vi "Agilent U2722 - Configure Chassis.vi"() -> ()   [LabVIEW 2018]
doc: "This VI shows how to configure chassis"
uses:
  <instrlib>/Agilent U2722/Agilent U2722.lvlib
panel:
  in  "Reference Clock Source (1: Auto)":i32(ring)=1 items=["Internal", "Auto"]
  in  "Trigger Out Bit (0)":i32
  in  "Chassis Identity (0)":i32
  in  "Chassis VISA resource name":refnum<visa-resource-name>
  # "(c) 2009-2015 National Instruments.  ALL RIGHTS RESERVED."
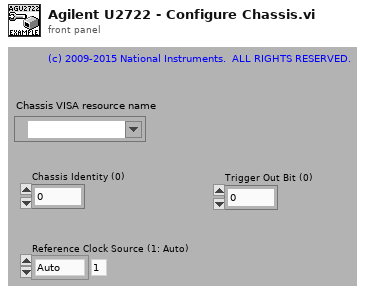
[diagram p1: front panel]
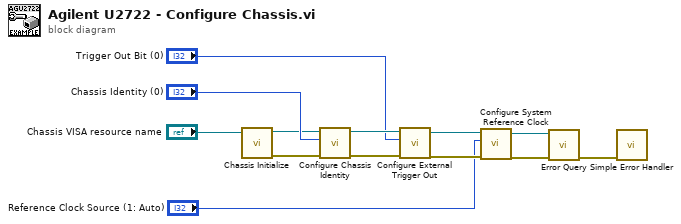
[diagram p0: block diagram]
diagram:
  n1 = call <instrlib>:"Chassis Initialize.vi"("Chassis VISA resource name"="Chassis VISA resource name") -> ("error out"=w2:errorcluster, "Chassis VISA resource name out"=w3:refnum<visa-resource-name>)  [unwired: 9 in]
  n2 = call <instrlib>:"Configure Chassis Identity.vi"("error in (no error)"=w2, "Chassis Identity (0)"="Chassis Identity (0)", "Chassis VISA resource name"=w3) -> ("error out"=w11:errorcluster, "Chassis VISA resource name out"=w9:refnum<visa-resource-name>)  [unwired: 7 in]
  n3 = call <instrlib>:"Configure External Trigger Out.vi"("error in (no error)"=w11, "Trigger Out Bit (0)"="Trigger Out Bit (0)", "Chassis VISA resource name"=w9) -> ("error out"=w12:errorcluster, "Chassis VISA resource name out"=w10:refnum<visa-resource-name>)  [unwired: 7 in]
  n4 = call <instrlib>:"Configure System Reference Clock.vi"("error in (no error)"=w12, "Reference Clock Source (1: Auto)"="Reference Clock Source (1: Auto)", "Chassis VISA resource name"=w10) -> ("error out"=w4:errorcluster, "Chassis VISA resource name out"=w5:refnum<visa-resource-name>)  [unwired: 7 in]
  n5 = call <instrlib>:"Error Query.vi"("error in (no error)"=w4, "VISA resource name"=w5) -> ("error out"=w13:errorcluster)  [unwired: 6 in, 3 out]
  n6 = call <vilib>:"Simple Error Handler.vi"("error in (no error)"=w13) -> ()  [unwired: 4 in, 5 out]
